vi "runtime to editor crosslink test.vi"() -> (0 "error out":errorcluster, 3 "Crosslinked?":bool)   [LabVIEW 2014, in "UI Reference tests.lvlib"]
uses:
  UI Reference tests.lvlib
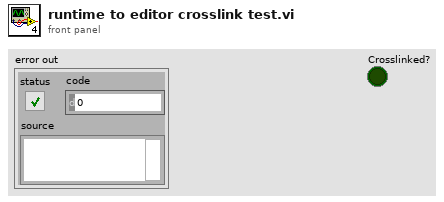
[diagram p1: front panel]
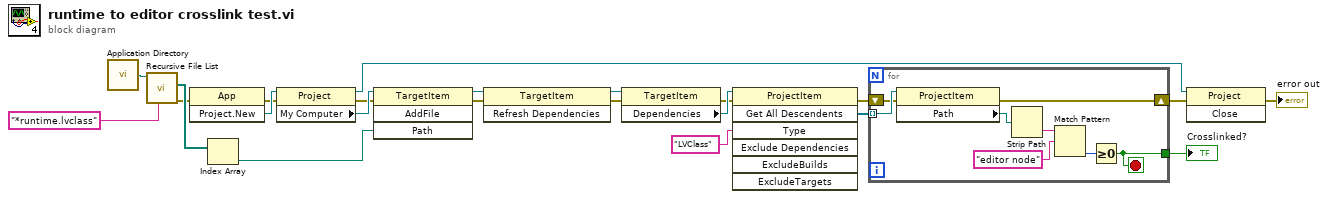
[diagram p0: block diagram]
diagram:
  n1 = call <vilib>:"Application Directory.vi"() -> ("Application Directory"=w5:path)
  n2 = call <vilib>:"Recursive File List.vi"("pattern"="*runtime.lvclass", "Folder Path"=w5) -> ("error out"=w1:errorcluster, "All Files in Dir"=w3:path[])  [unwired: 5 in, 3 out]
  n3 = invoke class="App" method="Project.New"(error in=w1) -> (error out=w16:errorcluster, "Project:New"=w19:refnum<vi>)  [unwired: 2 in, 1 out]
  n4 = Index Array(array=w3) -> (element=w2:path)  [unwired: 1 in]
  n5 = property class="Project"(reference=w19, error in=w16) -> (reference out=w10:refnum<vi>, error out=w17:errorcluster, "My Computer"=w18:refnum<vi>)
  n6 = invoke class="TargetItem" method="AddFile"(reference=w18, error in=w17, "Path"=w2) -> (reference out=w15:refnum<vi>, error out=w13:errorcluster)  [unwired: 1 in, 2 out]
  n7 = invoke class="TargetItem" method="Refresh Dependencies"(reference=w15, error in=w13) -> (reference out=w14:refnum<vi>, error out=w12:errorcluster)  [unwired: 1 in, 1 out]
  n8 = property class="TargetItem"(reference=w14, error in=w12) -> (error out=w8:errorcluster, "Dependencies"=w21:refnum<vi>)  [unwired: 1 out]
  n9 = invoke class="ProjectItem" method="Get All Descendents"(reference=w21, error in=w8, "Type"="LVClass") -> (error out=w9:errorcluster, "All Descendents"=w20:refnum<vi>[])  [unwired: 4 in, 5 out]
  n10 = for {
    tunnel: w20 -> [w30] mode=indexing
    shift-right: [w29] -> w11
    shift-left: w9 -> [w28]
    tunnel: [w23] -> w6
    stop <- w23 stop-if-true
    n11 = property class="ProjectItem"(reference=w30, error in=w28) -> (error out=w29:errorcluster, "Path"=w27:path)  [unwired: 1 out]
    n12 = Strip Path(path=w27) -> (name=w26:string)  [unwired: 1 out]
    n13 = Match Pattern(string=w26, regular expression="editor node") -> (offset past match=w24:i32)  [unwired: 1 in, 3 out]
    n14 = Greater Or Equal To 0?(x=w24) -> (x >= 0?=w23:bool)
  }
  "Crosslinked?" <- w6
  n15 = invoke class="Project" method="Close"(reference=w10, error in=w11) -> (error out=→"error out":errorcluster)  [unwired: 1 in, 2 out]
